vi "PXI_Host_I8_Write_OldMethod_Benchmark.vi"() -> ()   [LabVIEW 2018]
uses:
  <vilib>/Platform/TimedLoop/XDataNode/timing_clust.ctl
  <vilib>/Platform/TimedLoop/XDataNode/nitl_modes.ctl
  <vilib>/Platform/TimedLoop/XDataNode/wakeup.ctl
  <vilib>/NI/LVFPGA Adv Session Resources/OpenByNameSubVI.vi
  <vilib>/rvi/interface/common/dynamic/niFpgaEscapeDelimiterAndNull.vi
  <vilib>/Utility/error.llb/Error Cluster From Error Code.vi
  <vilib>/rvi/errors/niLvFpgaAdjustHostInterfaceError.vi
  <vilib>/FPGAPlugInAG/Dynamic/niLvFpga_Close_Dynamic.vi
  <vilib>/platform/TimedLoop/XDataNode/XDataNode.xnode
  <vilib>/NI/LVFPGA Adv Session Resources/OpenByName.xnode
  <vilib>/rvi/interface/nirviReadWriteControl/nirviReadWriteControl.xnode
  <vilib>/rvi/interface/nirviCloseFPGA/nirviCloseFPGA.xnode
  NiFpgaLv.dll
  <vilib>/rvi/interface/Simulation/niFpgaSimulationCallBeginRW.vi
  <vilib>/NI/LVFPGA Adv Session Resources/LVFPGAAdvSessionResources.lvlib
  cRIO RT/FPGA Bitfile Register Operations/Scalar IO Operations/FPGA Register IO.lvlib
  <vilib>/Platform/TimedLoop/XDataNode/XDNodeRunTimeDep.lvlib
panel:
  out "Maximum(s)":dbl
  out "Standard deviation":dbl
  out "Waveform Graph":dbl[](graph)
  out "error out":errorcluster
  out "Execution time (s)":dbl
  # "Recorded time"
  # "3.37551E-5"
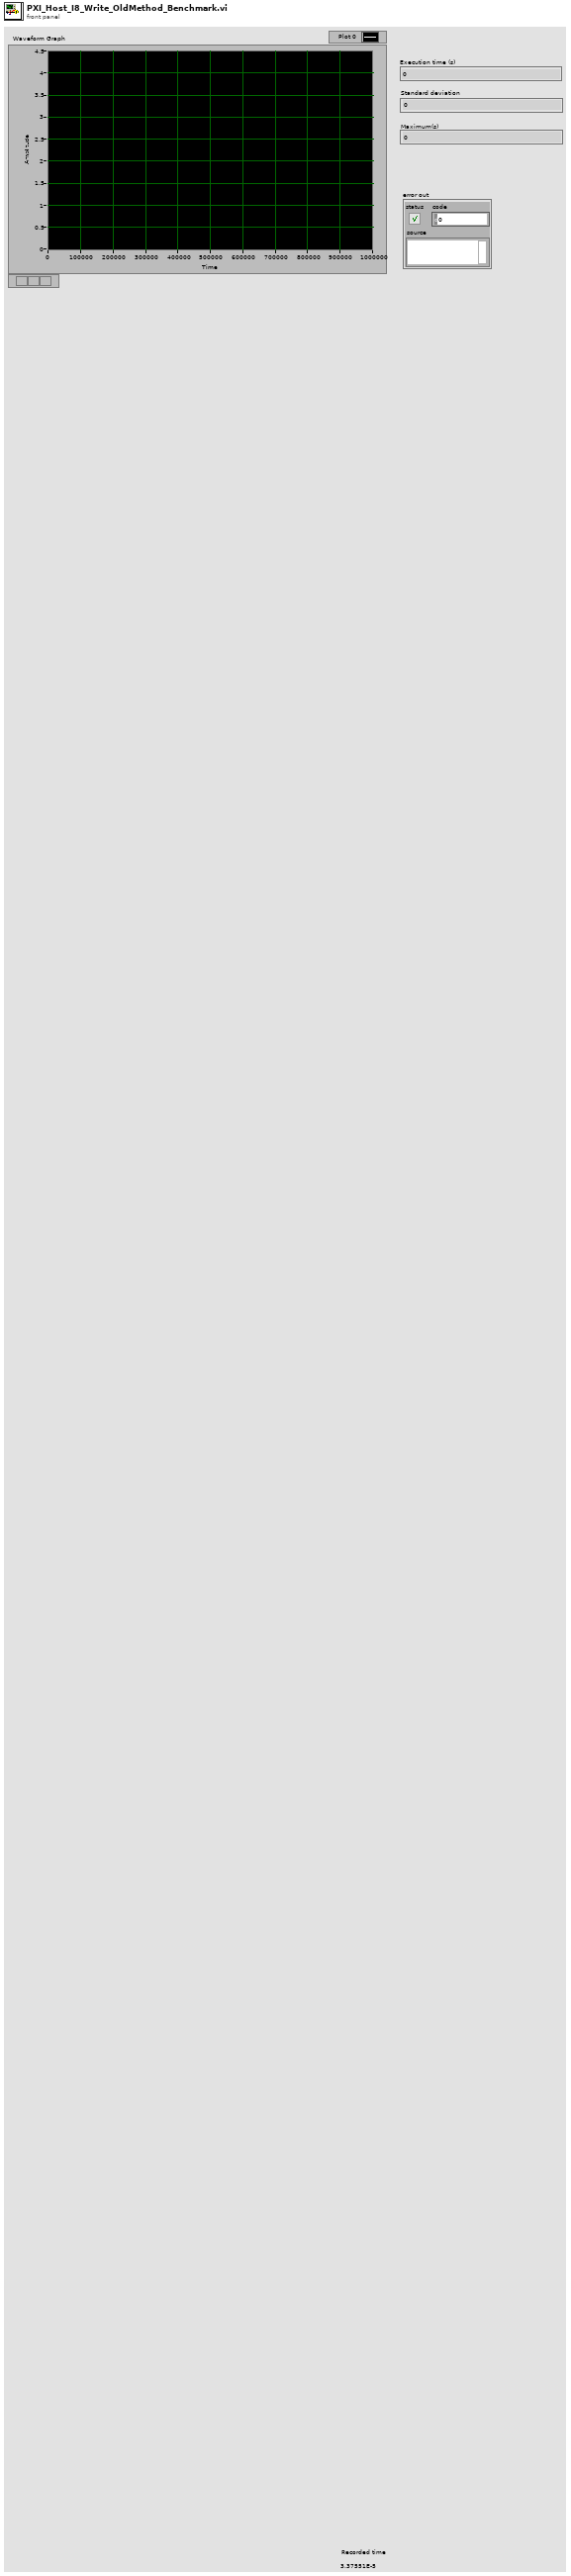
[diagram p1: front panel]
types:
  T1 = typedef "XDNodeRunTimeDep.lvlib/timing_clust.ctl" = cluster{"Expected End [f-1]":u64, "Actual End [f-1]":u64, "Finished Late? [f-1]":bool, "Expected End [i-1]":u64, "Actual End [i-1]":u64, "Finished Late? [i-1]":bool, "Expected Start [i]":u64, "Actual Start [i]":u64, "Expected Start [f]":u64, "Actual Start [f]":u64, "Source Name":string, "Structure Name":string, "Period":i64, "Deadline":i64, "Offset":i64, "Start":i64, "Priority":i32, "Timeout":i32, "Mode":T2, "Wakeup Reason":T3, "Error":errorcluster, "Source Type":string, "Secondary Source Type":string, "Global End Time":u64, "Global Start Time":u64, "Frame Duration":u64, "Iteration Duration":u64, "Assigned CPU":i32, "I/O Scan Engine Mode":u32}
  T2 = typedef "XDNodeRunTimeDep.lvlib/nitl_modes.ctl" = enum32{"No Change", "Process missed periods, maintain original phase", "Discard missed periods, maintain original phase", "Process missed periods, ignore original phase", "Discard missed periods, ignore original phase"}
  T3 = typedef "XDNodeRunTimeDep.lvlib/wakeup.ctl" = enum32{"Normal", "Aborted", "Asynchronous wakeup", "Timing source error", "Timed loop error", "Timeout"}
  T4 = cluster{"Name":string, "Depth":u32, "Write? (Deprecated:Use Implementation)":bool, "Physical Channel":u32, "Base Address":u32, "Data Width":u32, "Data Type":enum32{"Boolean", "I8", "I16", "I32", "I64", "U8", "U16", "U32", "U64", "FXP", "CustomControl", "SGL"}, "FXP Properties":variant, "Write Window Address":u32, "Implementation":enum16{"niFpgaTargetToHost", "niFpgaHostToTarget", "niFpgaPeerToPeerWriter", "niFpgaPeerToPeerReader", "niCoreTargetToHost", "niCoreHostToTarget"}, "Control Set":u32}[]
  T5 = cluster{"Name":string, "type":variant, "indicator?":bool}[]
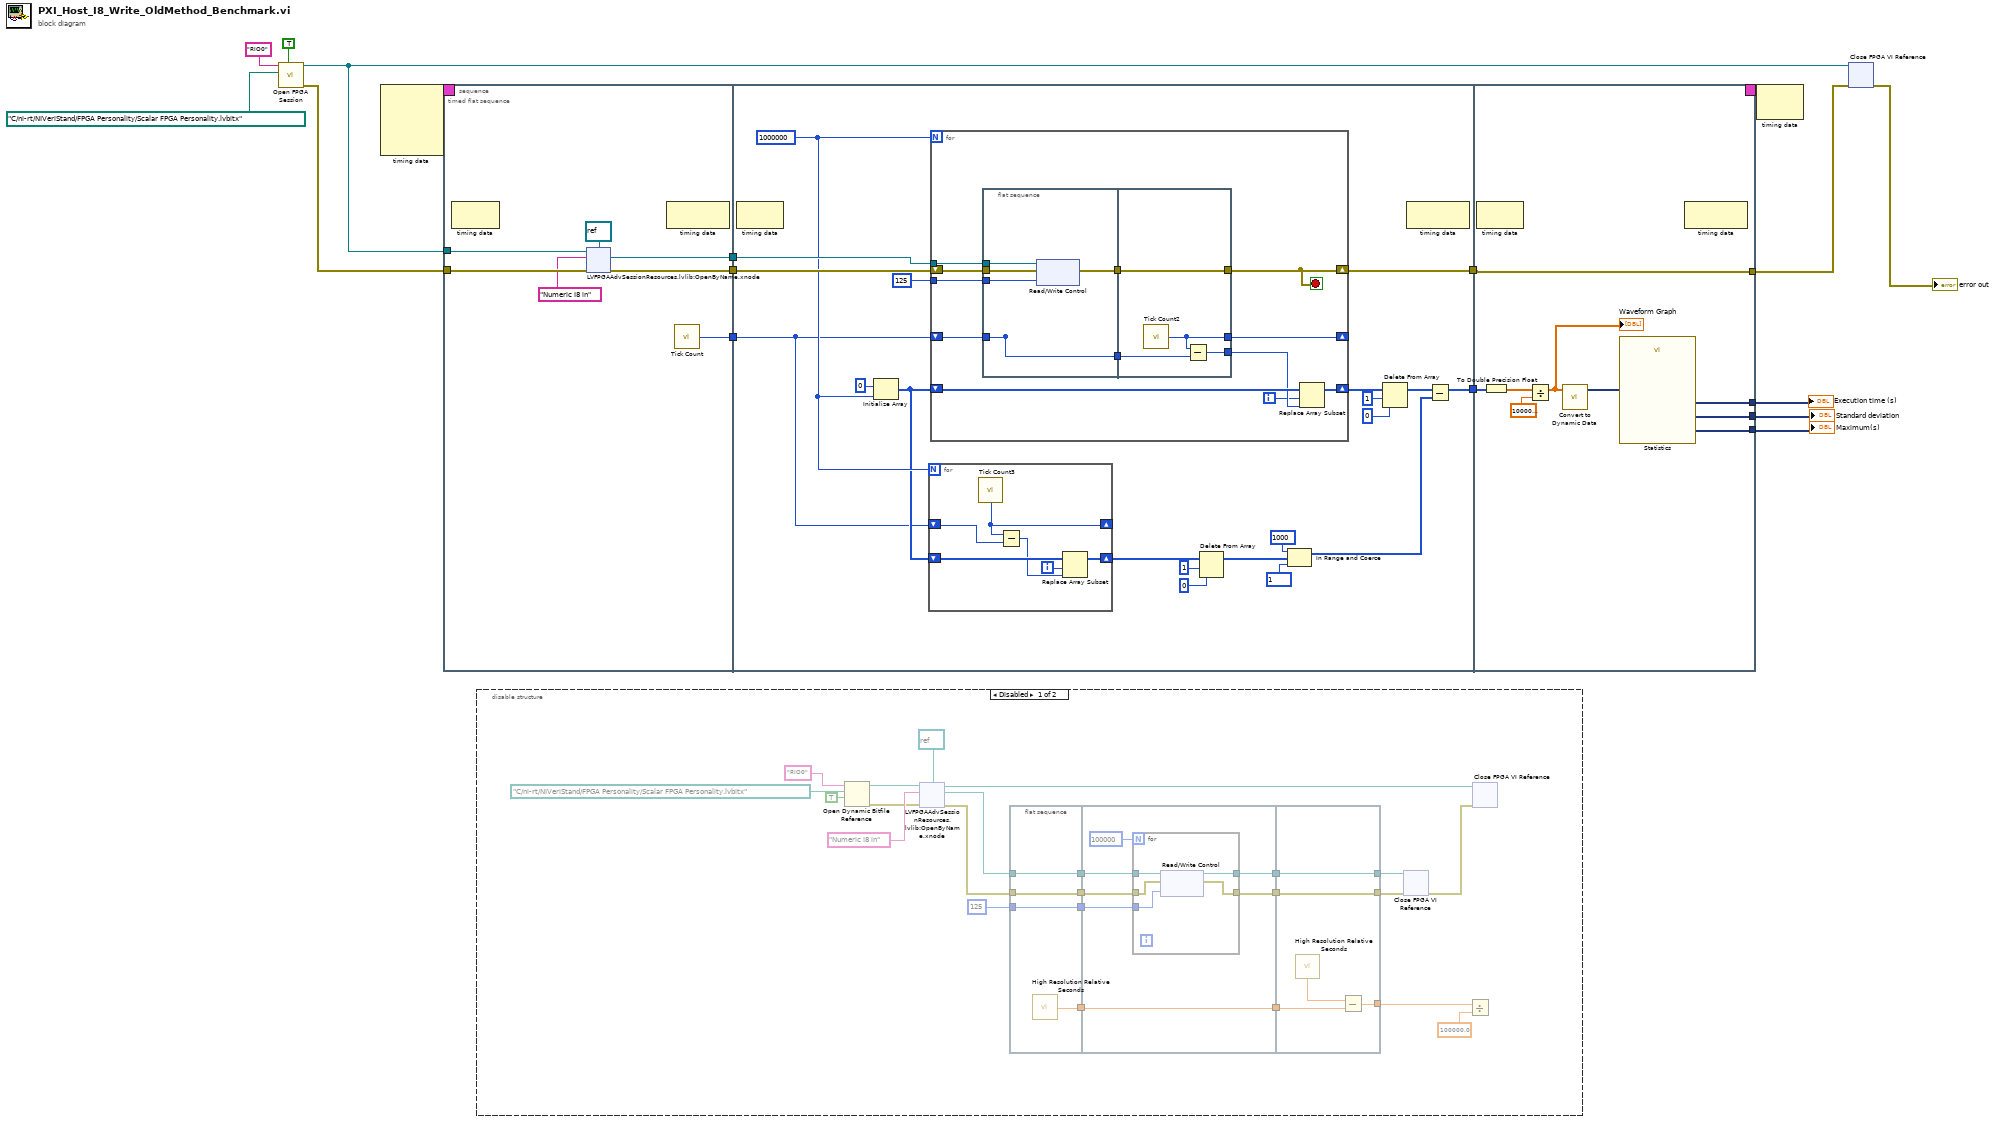
[diagram p0: block diagram]
diagram:
  n1 = call "Open FPGA Session.vi"("run when loaded (T)"=TRUE, "bitfile path"=path "C:/ni-rt/NIVeriStand/FPGA Personality/Scalar FPGA Personality.lvbitx", "device address"="RIO0") -> ("error out"=w7:errorcluster, "bitfile reference out"=w1:refnum<k20>)  [unwired: 6 in, 1 out]
  n2 = node-c288() -> (w12:T1)  [unwired: 4 in]
  n3 = timed-sequence {
    timing: w12 -> [_]
    timing-out: [_] -> w11
    tunnel: w7 -> [w14]
    tunnel: [w20] -> w6
    tunnel: [w17] -> w4
    tunnel: [w16] -> w3
    tunnel: [w15] -> w2
    tunnel: w1 -> [w13]
    n4 = timed-flat-sequence {
      tunnel: [w27] -> w23
      tunnel: [w28] -> w22
      tunnel: [w30] -> w19
      tunnel: w14 -> [w26]
      tunnel: w13 -> [w29]
      tunnel: w23 -> [w65]
      tunnel: [w64] -> w21
      tunnel: w22 -> [w63]
      tunnel: w19 -> [w54]
      tunnel: [w47] -> w18
      tunnel: w21 -> [w103]
      tunnel: [w103] -> w20
      tunnel: w18 -> [w96]
      tunnel: [w101] -> w17
      tunnel: [w99] -> w16
      tunnel: [w98] -> w15
      frame #0 {
        n5 = node-c288() -> ()  [unwired: 1 in, 1 out]
        n6 = xnode "LVFPGAAdvSessionResources.lvlib:OpenByName.xnode"("FPGA VI Reference in"=w29, "Resource name in"="Numeric I8 in", "Single resource reference type in"=refnum<k20> refnum ("Type"), "Error in"=w26) -> ("Single resource reference out"=w28:refnum<k20>, "Error out"=w27:errorcluster)  [unwired: 1 out]
        n7 = node-c288() -> ()  [unwired: 1 in, 1 out]
        n8 = call "Tick Count"() -> ("Tick Count(Ticks)"=w30:u32)
      }
      frame #1 {
        w56 = 1000000
        n9 = node-c288() -> ()  [unwired: 1 in, 1 out]
        n10 = Initialize Array(u32 0, w56) -> (w55:u32[])
        n11 = for {
          N: w56 -> [_]
          shift-right: [w66] -> w57
          shift-left: w55 -> [w69]
          shift-right: [w71] -> _
          shift-left: w54 -> [w70]
          i -> [w67]
          n12 = call "Tick Count3"() -> ("Tick Count(Ticks)"=w71:u32)
          n13 = Subtract(x=w71, y=w70) -> (x-y=w68:u32)
          n14 = Replace Array Subset(array=w69, new element=w68, index=w67) -> (w66:u32[])
        }
        n15 = for {
          N: w56 -> [_]
          tunnel: w63 -> [w84]
          shift-right: [w82] -> _
          shift-left: w54 -> [w81]
          shift-right: [w77] -> w61
          shift-left: w55 -> [w79]
          shift-right: [w75] -> w64
          shift-left: w65 -> [w85]
          tunnel: i8 125 ("Value") -> [w74]
          i -> [w76]
          stop <- w75 stop-if-true
          n16 = flat-sequence {
            tunnel: w85 -> [w89]
            tunnel: w84 -> [w87]
            tunnel: [w88] -> w83
            tunnel: [w90] -> _
            tunnel: w81 -> [w90]
            tunnel: [w90] -> w80
            tunnel: w74 -> [w86]
            tunnel: [w94] -> w75
            tunnel: w83 -> [w94]
            tunnel: [w93] -> w82
            tunnel: w80 -> [w92]
            tunnel: [w91] -> w78
            frame #0 {
              n17 = xnode "Read/Write Control"("FPGA VI Reference In"=w87, "error in"=w89, "Value"=w86) -> ("error out"=w88:errorcluster)  [unwired: 1 out]
            }
            frame #1 {
              n18 = call "Tick Count2"() -> ("Tick Count(Ticks)"=w93:u32)
              n19 = Subtract(x=w93, y=w92) -> (x-y=w91:u32)
            }
          }
          n20 = Replace Array Subset(array=w79, new element=w78, index=w76) -> (w77:u32[])
        }
        n21 = Delete From Array(array=w57, length=1, index=0) -> (array with subset deleted=w48:u32[])  [unwired: 1 out]
        n22 = In Range and Coerce(upper limit=u32 1000 ("Tick Count(Ticks)"), x=w48, lower limit=u32 1 ("Tick Count(Ticks)")) -> (coerced(x)=w49:u32[])  [unwired: 1 out]
        n23 = Delete From Array(array=w61, length=1, index=0) -> (array with subset deleted=w46:u32[])  [unwired: 1 out]
        n24 = node-c288() -> ()  [unwired: 1 in, 1 out]
        n25 = Subtract(x=w46, y=w49) -> (x-y=w47:u32[])
      }
      frame #2 {
        n26 = node-c288() -> ()  [unwired: 1 in, 1 out]
        n27 = To Double Precision Float(number=w96) -> (double precision float=w95:dbl[])
        n28 = Divide(x=w95, y=1000000000.0) -> (x/y=w97:dbl[])
        "Waveform Graph" <- w97
        n29 = call "Convert to Dynamic Data"("Array"=w97) -> ("Dynamic Data Type"=w102:dynamicdata)  [unwired: 3 in]
        n30 = call "Statistics"("Signals"=w102) -> ("Standard Dev"=w99:dynamicdata, "Arithmetic Mean"=w101:dynamicdata, "Maximum"=w98:dynamicdata)  [unwired: 23 in, 1 out]
        n31 = node-c288() -> ()  [unwired: 1 in, 1 out]
      }
    }
  }
  "Execution time (s)" <- w4
  "Standard deviation" <- w3
  "Maximum(s)" <- w2
  n32 = disable-structure shown="Disabled" {
    frame Disabled {
      n33 = Open Dynamic Bitfile Reference(0:"RIO0" ("Device address"), 1:path "C:/ni-rt/NIVeriStand/FPGA Personality/Scalar FPGA Personality.lvbitx" ("Bitfile path"), 2:TRUE ("Run When Loaded")) -> (5:w116:refnum<k20>, 8:w114:errorcluster)  [unwired: 2 in]
      n34 = xnode "LVFPGAAdvSessionResources.lvlib:OpenByName.xnode"("FPGA VI Reference in"=w116, "Resource name in"="Numeric I8 in", "Single resource reference type in"=refnum<k20> refnum ("Type"), "Error in"=w114) -> ("Single resource reference out"=w112:refnum<k20>, "Error out"=w113:errorcluster, "FPGA VI Reference out"=w109:refnum<k20>)
      n35 = flat-sequence {
        tunnel: [w132] -> w128
        tunnel: w112 -> [w131]
        tunnel: [w131] -> w127
        tunnel: [w130] -> w126
        tunnel: w113 -> [w130]
        tunnel: [w129] -> w125
        tunnel: i8 125 ("Value") -> [w129]
        tunnel: [w138] -> w124
        tunnel: w128 -> [w138]
        tunnel: w127 -> [w137]
        tunnel: w126 -> [w136]
        tunnel: [w135] -> w123
        tunnel: [w134] -> w122
        tunnel: w125 -> [w133]
        tunnel: w124 -> [w148]
        tunnel: [w147] -> w121
        tunnel: w123 -> [w146]
        tunnel: [w146] -> w108
        tunnel: w122 -> [w145]
        tunnel: [w145] -> w107
        frame #0 {
          n36 = call <vilib>:"High Resolution Relative Seconds.vi"() -> ("relative seconds"=w132:dbl)
        }
        frame #1 {
          n37 = for {
            N: 100000 -> [_]
            tunnel: w137 -> [w144]
            tunnel: w136 -> [w143]
            tunnel: [w142] -> w135
            tunnel: [w141] -> w134
            tunnel: w133 -> [w140]
            n38 = xnode "Read/Write Control"("FPGA VI Reference In"=w144, "error in"=w143, "Value"=w140) -> ("FPGA VI Reference Out"=w141:refnum<k20>, "error out"=w142:errorcluster)
          }
        }
        frame #2 {
          n39 = call <vilib>:"High Resolution Relative Seconds.vi"() -> ("relative seconds"=w149:dbl)
          n40 = Subtract(x=w149, y=w148) -> (x-y=w147:dbl)
        }
      }
      n41 = xnode "Close FPGA VI Reference"("FPGA VI Reference In"=w107, "error in"=w108) -> ("error out"=w110:errorcluster)
      n42 = Divide(x=w121, y=100000.0) -> ()  [unwired: 1 out]
      n43 = xnode "Close FPGA VI Reference"("FPGA VI Reference In"=w109, "error in"=w110) -> ()  [unwired: 1 out]
    }
    frame Enabled {
    }
  }
  n44 = node-c288(w11) -> ()  [unwired: 1 out]
  n45 = xnode "Close FPGA VI Reference"("FPGA VI Reference In"=w1, "error in"=w6) -> ("error out"=→"error out":errorcluster)
